vi "One Matching String Inputs.vi"(8 "error in (no error)":errorcluster, 11 "Mock in":refnum<class "Mock.lvclass">) -> (0 "error out":errorcluster, 3 "Mock out":refnum<class "Mock.lvclass">)   [LabVIEW 2020, in "Never.lvclass"]
uses:
  Framework/Mock/Mock.lvclass
  Comparators/Ignore Inputs Comparator/Ignore Inputs Comparator.lvclass
  C:/git/astemes-lmock/source/Core/Comparator/Comparator.lvclass
  Never.lvclass
  C:/git/astemes-lmock/source/Core/Expectation/Expectation.lvclass
  Never.lvclass/Never.ctl
  Comparators/String Argument Matching Comparator/String Input Matching Comparator.lvclass
  C:/git/astemes-lmock/source/Comparators/String Argument Matching Comparator/String Input Matching Comparator.lvclass
  C:/git/astemes-lmock/source/Expectations/Never/Never.lvclass
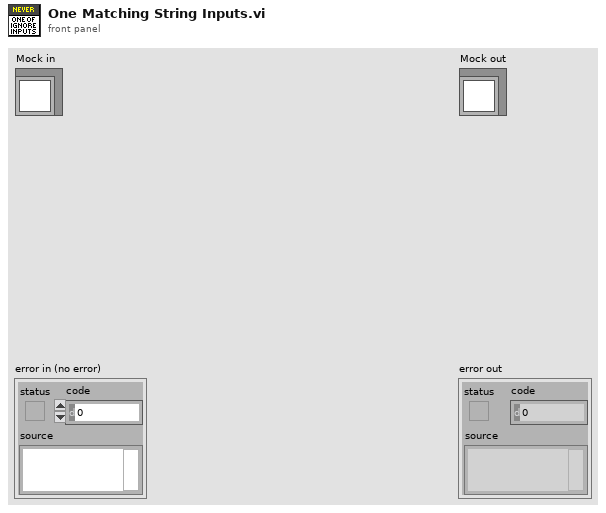
[diagram p1: front panel]
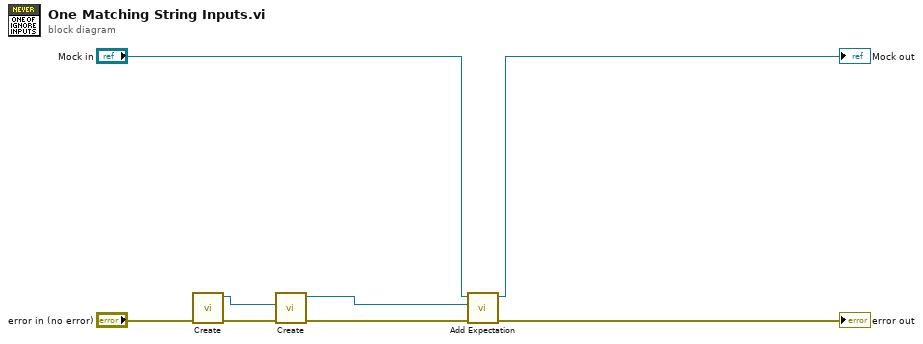
[diagram p0: block diagram]
diagram:
  n1 = call "Create.vi"("error in (no error)"="error in (no error)") -> ("error out"=w1:errorcluster, "String Argument Matching Comparator"=w3:refnum<class "String Input Matching Comparator.lvclass">)  [unwired: 9 in]
  n2 = call "Create.vi"("error in (no error)"=w1, "Comparator"=w3) -> ("error out"=w5:errorcluster, "One"=w4:refnum<class "Never.lvclass">)  [unwired: 8 in]
  n3 = call-dynamic "Add Expectation.vi"("error in (no error)"=w5, "Expectations"=w4, "Mock in"="Mock in") -> ("error out"=→"error out":errorcluster, "Mock out"=→"Mock out":refnum<class "Mock.lvclass">)  [unwired: 7 in]
